vi "Tag AE.vi"(6 "Persistence":bool, 7 "Mode":T1(ring), 8 "错误输入（无错误）":errorcluster, 9 "Tag Value In":variant, 10 "Tag Name":string, 11 "Ctl Ref In":refnum<vi>) -> (0 "错误输出":errorcluster, 1 "Tag Value Out":variant, 2 "Succeed?":bool, 3 "Ctl Ref Out":refnum<vi>, 4 "Persistence?":bool)   [LabVIEW 2012, in "CtrlRef.lvlib"]
uses:
  CtrlRef.lvlib
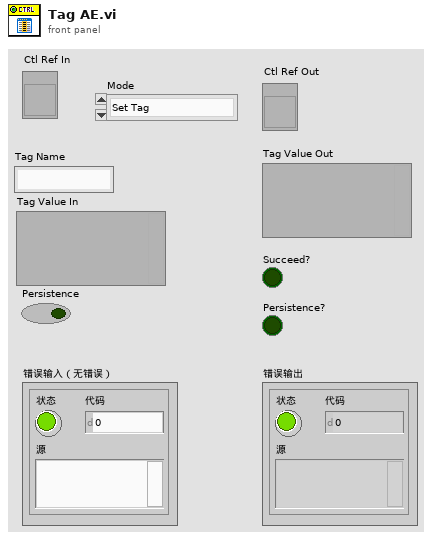
[diagram p1: front panel]
types:
  T1 = enum16{"Set Tag", "Get Tag", "Remove Tag", "Set Tag Persistence"}
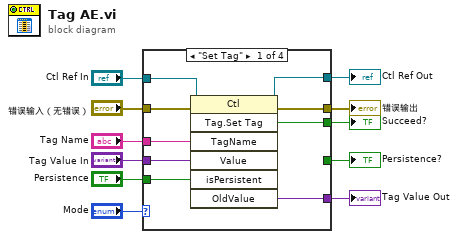
[diagram p0: block diagram]
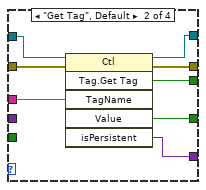
[diagram p2: hidden frame]
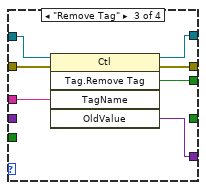
[diagram p3: hidden frame]
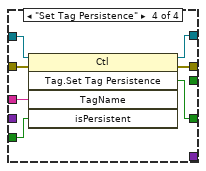
[diagram p4: hidden frame]
diagram:
  n1 = case shown="\"Set Tag\"" "Mode" {
    tunnel: "Ctl Ref In" -> [w20 w28 w35 w38]
    tunnel: [w19 w27 w34 w37] -> w9
    tunnel: "Tag Name" -> [w16 w26 w32 w41]
    tunnel: [_ w25 _ w40] -> w7
    tunnel: [w12 w24 w33 _] -> w6
    tunnel: [w14 w23 w31 _] -> w5
    tunnel: "错误输入（无错误）" -> [w18 w22 w30 w39]
    tunnel: [w17 w21 w29 w36] -> w3
    tunnel: "Tag Value In" -> [w15 _ _ _]
    tunnel: "Persistence" -> [w13 _ _ w42]
    frame "Set Tag" {
      n2 = invoke class="Ctl" method="Tag.Set Tag"(reference=w20, error in=w18, "TagName"=w16, "Value"=w15, "isPersistent"=w13) -> (reference out=w19:refnum<vi>, error out=w17:errorcluster, "SetTag"=w12:bool, "OldValue"=w14:variant)  [unwired: 2 in, 3 out]
    }
    frame "Get Tag", Default {
      n3 = invoke class="Ctl" method="Tag.Get Tag"(reference=w28, error in=w22, "TagName"=w26) -> (reference out=w27:refnum<vi>, error out=w21:errorcluster, "GetTag"=w24:bool, "Value"=w25:bool, "isPersistent"=w23:variant)  [unwired: 3 in, 1 out]
    }
    frame "Remove Tag" {
      n4 = invoke class="Ctl" method="Tag.Remove Tag"(reference=w35, error in=w30, "TagName"=w32) -> (reference out=w34:refnum<vi>, error out=w29:errorcluster, "RemoveTag"=w33:bool, "OldValue"=w31:variant)  [unwired: 2 in, 1 out]
    }
    frame "Set Tag Persistence" {
      n5 = invoke class="Ctl" method="Tag.Set Tag Persistence"(reference=w38, error in=w39, "TagName"=w41, "isPersistent"=w42) -> (reference out=w37:refnum<vi>, error out=w36:errorcluster, "SetTagPersistence"=w40:bool)  [unwired: 1 in, 2 out]
    }
  }
  "Ctl Ref Out" <- w9
  "错误输出" <- w3
  "Persistence?" <- w7
  "Succeed?" <- w6
  "Tag Value Out" <- w5
